vi "Create Log Header String.vi"(8 "error in (no error)":errorcluster, 11 "LogEngine in":refnum<class "LogEngine.lvclass">) -> (0 "error out":errorcluster, 2 "LogHeaderString":string, 3 "LogEngine out":refnum<class "LogEngine.lvclass">)   [LabVIEW 2017, in "LogEngine.lvclass"]
doc: "Developed by Kevin Thompson\nkevin@thompsonengineering.net\n\nCopyright 2018-2020\nThompson Engineering, LLC"
uses:
  LogEngine.lvclass
  Accessors/Get ObjData.vi
  Accessors/Set ObjData.vi
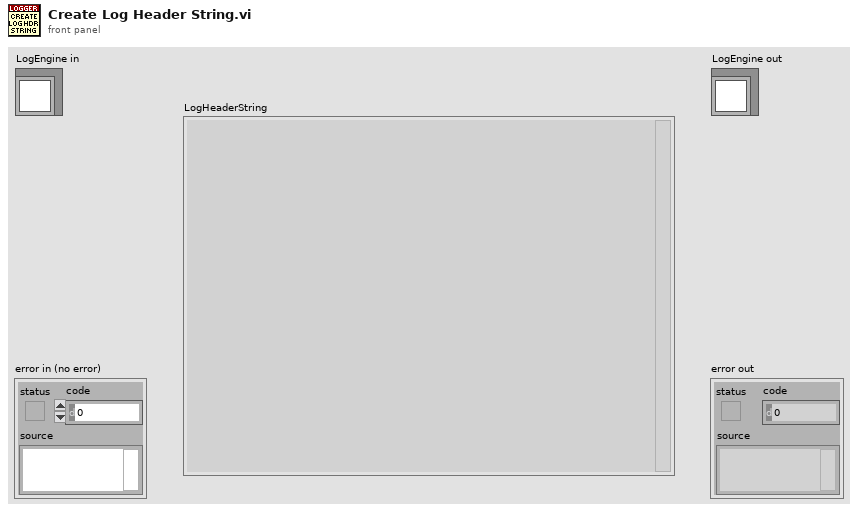
[diagram p1: front panel]
types:
  T1 = typedef "LogEngine.lvclass/TD Obj Data_LogEngine.ctl" = cluster{"LogEngine Settings":T2, "Logger State Data":T3, "tdms fileref":refnum<k34>, "LogHeaderData":T5, "LogHeaderString":string}
  T2 = typedef "LogEngine.lvclass/TD LogEngine Settings--cluster.ctl" = cluster{"placeholder":string, "LogWriteIntv (ms)":u32, "LogFile folder name":string, "TDMS folder name":string}
  T3 = typedef "LogEngine.lvclass/TD Logger State Data--cluster.ctl" = cluster{"Logger State":T4, "TDMS Logging State":T4, "LogFile path":path, "TDMS File path":path, "vData":variant}
  T4 = typedef "LogEngine.lvclass/TD Logger State--enum.ctl" = enum16{"Unknown", "Logging", "NotLogging", "Error"}
  T5 = typedef "LogEngine.lvclass/LogHeaderData--cluster.ctl" = cluster{"SessionSettings":T6, "SequenceFile":string, "Curr_WeldCount":i32, "SeqFileParams":T7, "AI TaskName":string, "SamplingRate":dbl, "SamplesPerAcq":i32}
  T6 = typedef "SessionSettings--cluster.ctl" = cluster{"Job_ID":string, "Operator_ID":string, "Station_ID":string, "Job_Description":string}
  T7 = typedef "Sequencer.lvclass/SeqFileParameters--cluster.ctl" = cluster{"MotorVel":dbl, "VoltageSP":dbl, "MoveSF":dbl, "IntegTime":dbl, "Pgain":dbl, "Igain":dbl, "Dgain":dbl, "PosMode":T8, "OscMode":T9, "WeldCurSF":dbl}
  T8 = typedef "Sequencer.lvclass/SeqFileParam_PosMode--enum.ctl" = enum16{"NORM", "ABS", "HYBRID"}
  T9 = typedef "Sequencer.lvclass/SeqFileParam_OscMode--enum.ctl" = enum16{"OFF", "ON"}
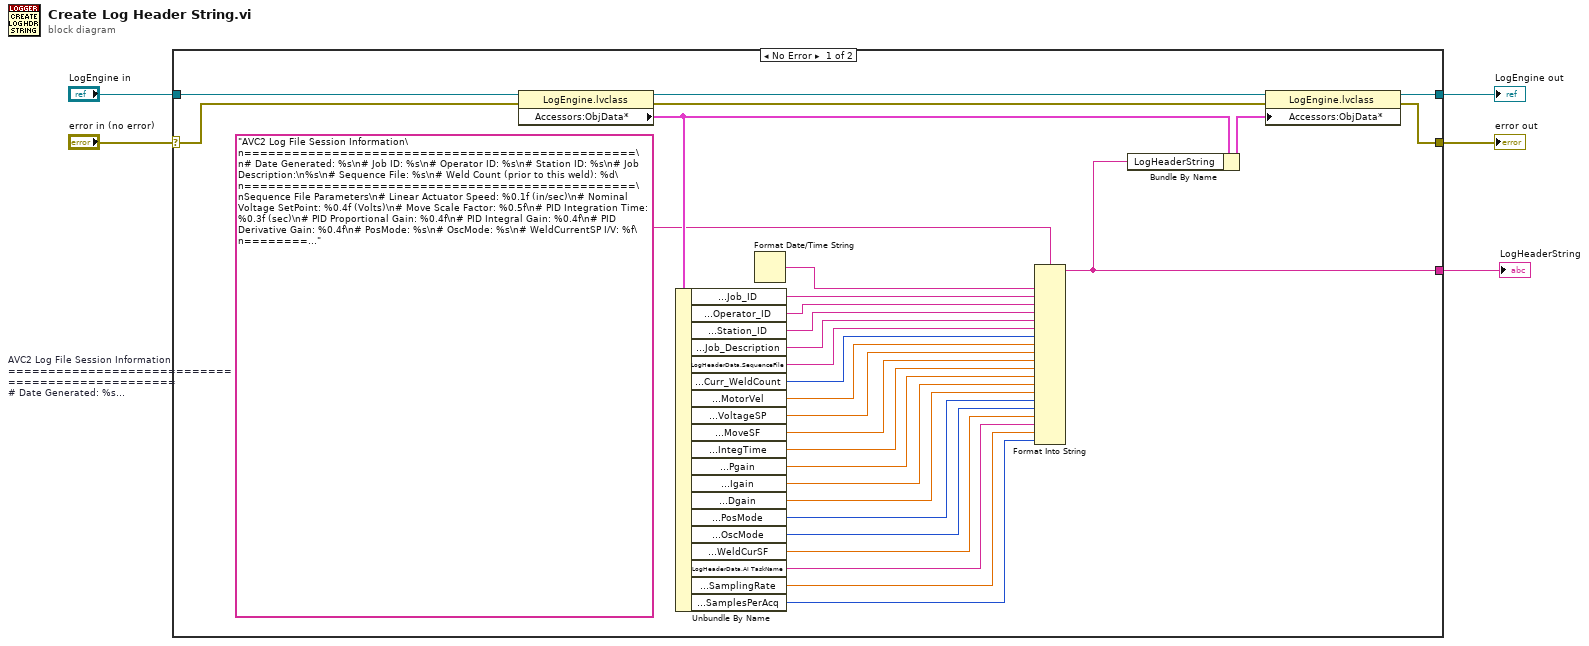
[diagram p0: block diagram]
diagram:
  n1 = case shown="No Error" "error in (no error)" {
    selector: "error in (no error)" -> [w21 w37]
    tunnel: [w20 w37] -> w4
    tunnel: [w27 w36] -> w2
    tunnel: "LogEngine in" -> [w35 w36]
    tunnel: [w25 _] -> w1
    frame No Error {
      w23 = "AVC2 Log File Session Information\n=================================================\n# Date Generated: %s\n# Job ID: %s\n# Operator ID: %s\n# Station ID: %s\n# Job Description:\n%s\n# Sequence File: %s\n# Weld Count (prior to this weld): %d\n=================================================\nSequence File Parameters\n# Linear Actuator Speed: %0.1f (in/sec)\n# Nominal Voltage SetPoint: %0.4f (Volts)\n# Move Scale Factor: %0.5f\n# PID Integration Time: %0.3f (sec)\n# PID Proportional Gain: %0.4f\n# PID Integral Gain: %0.4f\n# PID Derivative Gain: %0.4f\n# PosMode: %s\n# OscMode: %s\n# WeldCurrentSP I/V: %f\n=================================================\n# AI TaskName: %s\n# AI Sampling Rate: %0.1f (Samples Per Sec)\n# AI Samples Per Acq: %d\n=================================================\n\nTimestamp,RecTS,StepNum,WeldCurrent(A),VoltageDyn(V),CurrentDyn(A),VSPSum(V),PID_VError(V),PID_Pval,PID_Dval,PID_Ival,IDerror,TotalCtlrGain(V),TotalMove(mil),AVCLockout\n"  # AVC2 Log File Session Information ================================================= # Date Generated: %s # Job ID: %s # Operator ID: %s # Station ID: %s # Job Description: %s # Sequence File: %s # Weld Count (prior to this weld): %d ================================================= Sequence File Parameters # Linear Actuator Speed: %0.1f (in/sec) # Nominal Voltage SetPoint: %0.4f (Volts) # Move Scale Factor: %0.5f # PID Integration Time: %0.3f (sec) # PID Proportional Gain: %0.4f # PID Integral Gain: %0.4f # PID Derivative Gain: %0.4f # PosMode: %s # OscMode: %s # WeldCurrentSP I/V: %f ================================================= # AI TaskName: %s # AI Sampling Rate: %0.1f (Samples Per Sec) # AI Samples Per Acq: %d =================================================  Timestamp,RecTS,StepNum,WeldCurrent(A),VoltageDyn(V),CurrentDyn(A),VSPSum(V),PID_VError(V),PID_Pval,PID_Dval,PID_Ival,IDerror,TotalCtlrGain(V),TotalMove(mil),AVCLockout
      n2 = property class="LogEngine.lvclass"(reference=w35, error in=w21) -> (reference out=w34:refnum<class "LogEngine.lvclass">, error out=w22:errorcluster, "Accessors:ObjData*"=w24:T1)
      n3 = Unbundle By Name(w24) -> ("LogHeaderData.SessionSettings.Job_ID"=w33:string, "LogHeaderData.SessionSettings.Operator_ID"=w32:string, "LogHeaderData.SessionSettings.Station_ID"=w31:string, "LogHeaderData.SessionSettings.Job_Description"=w30:string, "LogHeaderData.SequenceFile"=w29:string, "LogHeaderData.Curr_WeldCount"=w6:i32, "LogHeaderData.SeqFileParams.MotorVel"=w7:dbl, "LogHeaderData.SeqFileParams.VoltageSP"=w8:dbl, "LogHeaderData.SeqFileParams.MoveSF"=w9:dbl, "LogHeaderData.SeqFileParams.IntegTime"=w10:dbl, "LogHeaderData.SeqFileParams.Pgain"=w11:dbl, "LogHeaderData.SeqFileParams.Igain"=w12:dbl, "LogHeaderData.SeqFileParams.Dgain"=w13:dbl, "LogHeaderData.SeqFileParams.PosMode"=w14:T8, "LogHeaderData.SeqFileParams.OscMode"=w15:T9, "LogHeaderData.SeqFileParams.WeldCurSF"=w16:dbl, "LogHeaderData.AI TaskName"=w17:string, "LogHeaderData.SamplingRate"=w18:dbl, "LogHeaderData.SamplesPerAcq"=w19:i32)
      n4 = Format Date/Time String() -> (date/time string=w28:string)  [unwired: 3 in]
      n5 = Format Into String(format string=w23, w28, w33, w32, w31, w30, w29, w6, w7, w8, w9, w10, w11, w12, w13, w14, w15, w16, w17, w18, w19) -> (resulting string=w25:string)  [unwired: 2 in, 1 out]
      n6 = Bundle By Name(cluster=w24, "LogHeaderString"=w25) -> (w26:T1)
      n7 = property class="LogEngine.lvclass"(reference=w34, error in=w22, "Accessors:ObjData*"=w26) -> (reference out=w27:refnum<class "LogEngine.lvclass">, error out=w20:errorcluster)
    }
    frame Error {
    }
  }
  "error out" <- w4
  "LogEngine out" <- w2
  "LogHeaderString" <- w1
